vi "Wolna_GET_ATTR.vi"(8 "error in (no error)":errorcluster, 11 "Wolna in":waveform(dbl)) -> (0 "error out":errorcluster, 3 "Wolna out":waveform(dbl), 4 "Typ rejestracji":T1, 5 "Kanaly":i32[](array[numeric]))   [LabVIEW 2013]
doc: "Pobiera atrybuty z waveforma rejestracji wolnej\nPobierane atrybuty: Typ_Rejestracji, Kanaly"
uses:
  Kontrolki/GUI/RejWol_typ.ctl
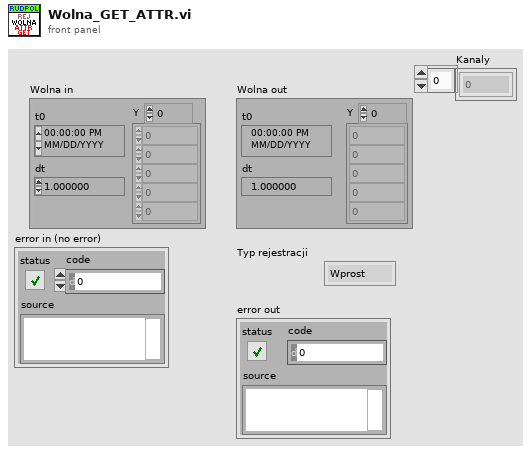
[diagram p1: front panel]
types:
  T1 = typedef "RejWol_typ.ctl" = enum16{"Wprost", "Moduł", "Kwadrat", "Iloczyn", "Faza"}
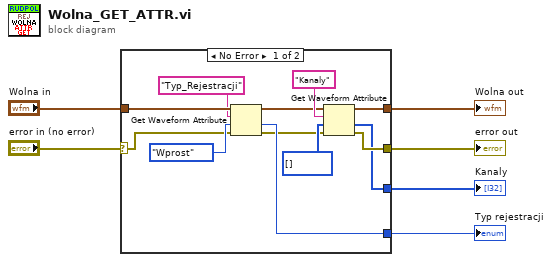
[diagram p0: block diagram]
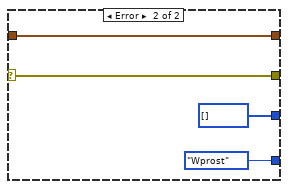
[diagram p2: hidden frame]
diagram:
  n1 = case shown="No Error" "error in (no error)" {
    selector: "error in (no error)" -> [w7 w20]
    tunnel: "Wolna in" -> [w18 w19]
    tunnel: [w17 RejWol_typ."Wprost" ("Typ rejestracji")] -> w5
    tunnel: [w12 w19] -> w4
    tunnel: [w9 w20] -> w3
    tunnel: [w8 i32[] [] ("Rejestracja wolna.Rej.2.Kanały")] -> w2
    frame No Error {
      n2 = Get Waveform Attribute(4:w7, 5:RejWol_typ."Wprost" ("Typ rejestracji"), 6:"Typ_Rejestracji", 7:w18) -> (0:w10:errorcluster, 1:w17:T1, 3:w13:waveform(dbl))  [unwired: 1 out]
      n3 = Get Waveform Attribute(4:w10, 5:i32[] [] ("Rejestracja wolna.Rej.2.Kanały"), 6:"Kanaly", 7:w13) -> (0:w9:errorcluster, 1:w8:i32[], 3:w12:waveform(dbl))  [unwired: 1 out]
    }
    frame Error {
    }
  }
  "error out" <- w3
  "Wolna out" <- w4
  "Typ rejestracji" <- w5
  "Kanaly" <- w2
